vi "uActor_CMDs_Prefix.vi"(1 "uActor CMD":string) -> (0 "Reserved CMD":string)   [LabVIEW 2023, in "uLib.lvlib" / "uActor.lvclass"]
doc: "Reserved CMDs are a special combination of a class specific command and a UUID+ClassName to prevent name/string collisions across the actor inheritance chain.\nEvery reserved command is either associated with a dynamic dispatch 'core' method or a special statically linked API VI. The reserved full command string is not exposed outside of this class and cannot be overriden by the children unless there is a special dynamic dispatch method for that. They cannot be overriden by using the EXEC method's case structure."
uses:
  uActor.lvclass
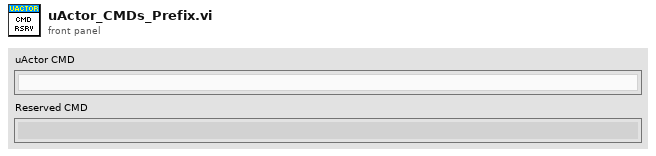
[diagram p1: front panel]
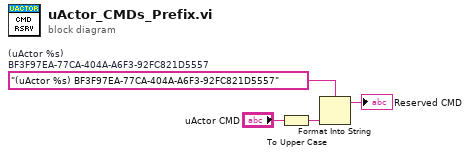
[diagram p0: block diagram]
diagram:
  w4 = "(uActor %s) BF3F97EA-77CA-404A-A6F3-92FC821D5557"  # (uActor %s) BF3F97EA-77CA-404A-A6F3-92FC821D5557
  n1 = To Upper Case(1:"uActor CMD") -> (0:w1:string)
  n2 = Format Into String(format string=w4, w1) -> (resulting string=→"Reserved CMD":string)  [unwired: 2 in, 1 out]
